vi "FunctDataMgr.Add Local SW Items.vi"(7 "Init(T)/Append(F)":bool, 8 "error in (no error)":errorcluster, 10 "Local SW Items":T1[](array[typedef]), 11 "FunctDataMgr in":refnum<class "FunctDataMgr.lvclass">) -> (0 "error out":errorcluster, 3 "FunctDataMgr":refnum<class "FunctDataMgr.lvclass">)   [LabVIEW 2018, in "FunctDataMgr.lvclass"]
uses:
  FunctDataMgr.lvclass
  Results/Result XML/TestResult.SW Item.ctl
  FunctDataMgr.lvclass/FunctDataMgr.ctl
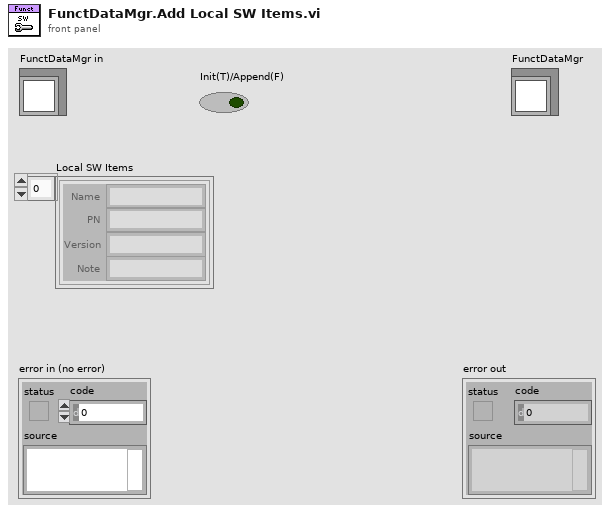
[diagram p1: front panel]
types:
  T1 = typedef "TestResult.SW Item.ctl" = cluster{"Name":string, "PN":string, "Version":string, "Note":string}
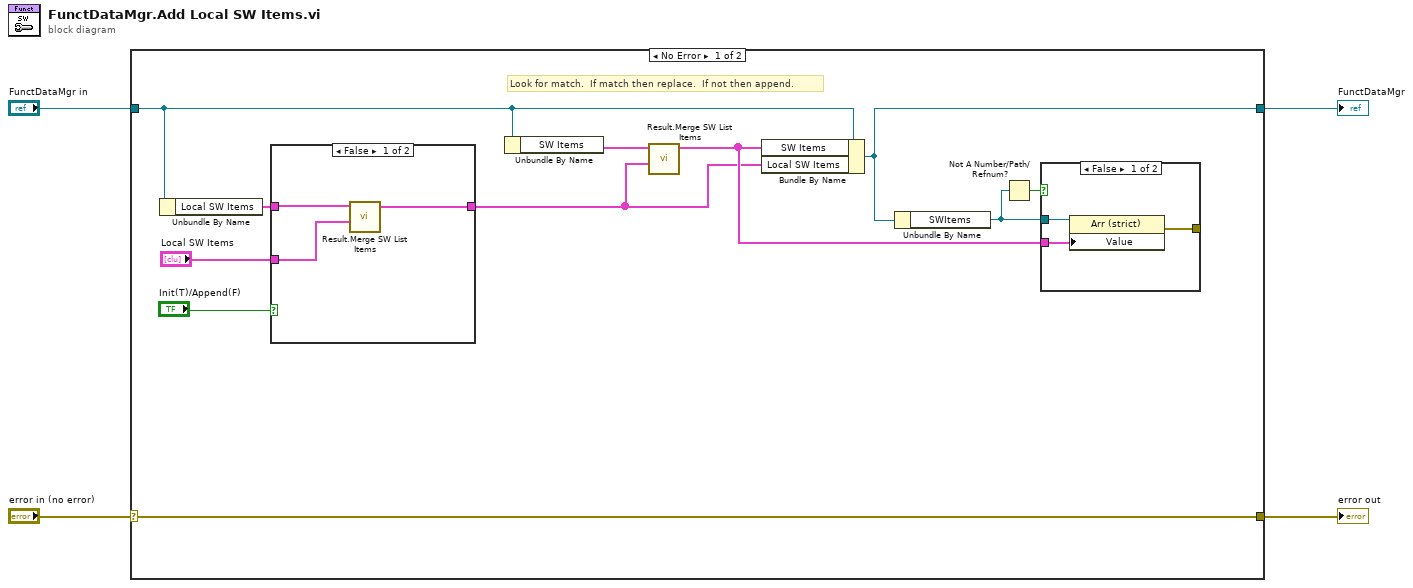
[diagram p0: block diagram]
diagram:
  n1 = case shown="No Error" "error in (no error)" {
    selector: "error in (no error)" -> [w15 w24]
    tunnel: [w15 w24] -> w3
    tunnel: [w8 w23] -> w1
    tunnel: "FunctDataMgr in" -> [w9 w23]
    frame No Error {
      # "Look for match.  If match then replace.  If not then append."
      n2 = Unbundle By Name(w9) -> ("Local SW Items"=w12:T1[])
      n3 = case shown="False" "Init(T)/Append(F)" {
        tunnel: "Local SW Items" -> [w20 w22]
        tunnel: w12 -> [w21 _]
        tunnel: [w19 w22] -> w5
        frame False {
          n4 = call "Result.Merge SW List Items.vi"("Old Items"=w20, "New Items"=w21) -> ("Merged Items"=w19:T1[])  [unwired: 9 in]
        }
        frame True {
        }
      }
      n5 = Unbundle By Name(w9) -> ("SW Items"=w7:T1[])
      n6 = call "Result.Merge SW List Items.vi"("Old Items"=w5, "New Items"=w7) -> ("Merged Items"=w6:T1[])  [unwired: 9 in]
      n7 = Bundle By Name(cluster=w9, "SW Items"=w6, "Local SW Items"=w5) -> (w8:refnum<class "FunctDataMgr.lvclass">)
      n8 = Unbundle By Name(w8) -> ("SWItems"=w11:refnum<vi>)
      n9 = Not A Number/Path/Refnum?(number/path/refnum=w11) -> (NaN/Path/Refnum?=w10:bool)
      n10 = case shown="False" w10 {
        tunnel: w11 -> [w18 _]
        tunnel: w6 -> [w17 _]
        tunnel: [w16 _] -> _
        frame False {
          n11 = property class="Arr (strict)"(reference=w18, "Value"=w17) -> (error out=w16:errorcluster)  [unwired: 1 in, 1 out]
        }
        frame True {
        }
      }
    }
    frame Error {
    }
  }
  "error out" <- w3
  "FunctDataMgr" <- w1
